vi "Configure OVP.vi"(7 "Limit (0.0 volts)":dbl format="%^.3e", 8 "error in (no error)":errorcluster {"code" format="%.0x"}, 9 "OVP Enabled (True)":bool=TRUE, 10 "Channel Name (1)":string="1", 11 "VISA resource name":refnum<visa-resource-name>) -> (0 "error out":errorcluster {"code" format="%.0x"}, 3 "VISA resource name out":refnum<visa-resource-name>)   [LabVIEW 2010, in "Agilent N6700 Series.lvlib"]
doc: "This VI configures the power supply's over-voltage protection. You specifies the over-voltage limit and the behavior of the power supply when the output voltage is greater than or equal to that value.\n\nWhen the enabled parameter is FALSE, the driver ignores the limit parameter and does not set the agn6700>>Basic Operation>>OVP Limit property.\n\n<B>Note: </B>\nThis VI has been obsoleted from the driver and is included for compatibility with existing applications. <B> New applications should use the Configure Over Voltage Protection VI</B>\n\nThe Agilent N6700 DC Power Supply is not allowed to enable/disable OVP."
uses:
  Agilent N6700 Series.lvlib
panel:
  # "Note:\nThis VI has been obsoleted from the driver and is included for compatibility with existing applications.  New applications should use the Configure Over Voltage Protection VI"
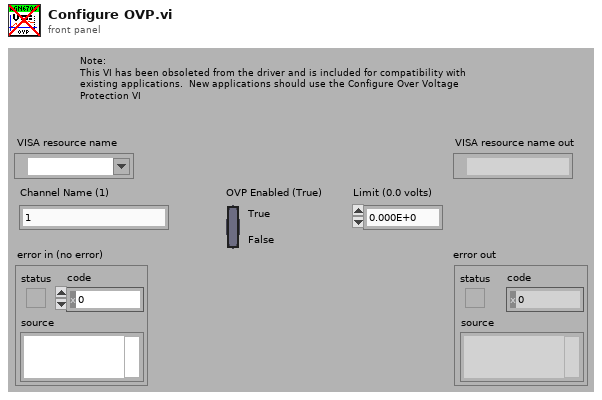
[diagram p1: front panel]
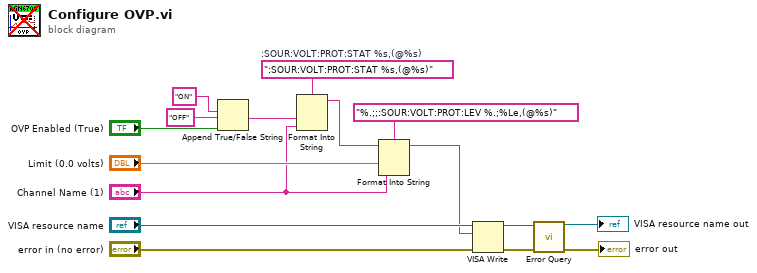
[diagram p0: block diagram]
diagram:
  w15 = ":SOUR:VOLT:PROT:STAT %s,(@%s)"  # :SOUR:VOLT:PROT:STAT %s,(@%s)
  n1 = Append True/False String(1:"OVP Enabled (True)", 2:"OFF", 3:"ON") -> (0:w8:string)  [unwired: 1 in]
  n2 = Format Into String(format string=w15, w8, "Channel Name (1)") -> (resulting string=w7:string)  [unwired: 2 in, 1 out]
  n3 = Format Into String(format string="%.;;:SOUR:VOLT:PROT:LEV %.;%Le,(@%s)", initial string=w7, "Limit (0.0 volts)", "Channel Name (1)") -> (resulting string=w5:string)  [unwired: 1 in, 1 out]
  n4 = VISA Write(VISA resource name="VISA resource name", write buffer=w5, error in (no error)="error in (no error)") -> (VISA resource name out=w2:refnum<visa-resource-name>, error out=w1:errorcluster)  [unwired: 1 out]
  n5 = call "Error Query.vi"("VISA resource name"=w2, "error in (no error)"=w1) -> ("VISA resource name out"=→"VISA resource name out":refnum<visa-resource-name>, "error out"=→"error out":errorcluster)  [unwired: 10 in, 2 out]
